vi "比较x与x+100.vi"() -> ()   [LabVIEW 2020]
panel:
  out "布尔":bool=TRUE
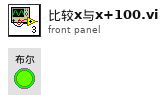
[diagram p1: front panel]
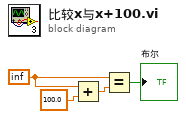
[diagram p0: block diagram]
diagram:
  w4 = inf
  n1 = Add(x=w4, y=100.0) -> (x+y=w2:dbl)
  n2 = Equal?(x=w4, y=w2) -> (x = y?=→"布尔":bool)
